vi "Smart_arm_Labview.vi"() -> ()   [LabVIEW 2022 SP3]
uses:
  <vilib>/Instr/_visa.llb/VISA Configure Serial Port (Instr).vi
panel:
  out "Number_of_runs":i16
  out "Stopped":bool
  out "Running":bool
  out "Read Target":string
  in  "Byte":u32
  in  "Joint 2":u8(knob) scale=45.0..100.0
  in  "Joint 1":u8(knob) scale=40.0..140.0
  in  "Buttom":u8(knob) scale=50.0..150.0
  out "Selected Mode":string
  in  "Mode_Selection":u8=1 max=2 step=1
  in  "Message Arduino -  Mode":bool
  in  "Claw":bool
  out "Previous settings of Claw, Buttom, Joint1, Joint2:":string
  in  "?":bool
  in  "Message Arduino - Angles":bool
  # "Smart Robotic Arm Control Panel"
  # "Automatic Mode"
  # "Select Mode"
  # "Hybrid Mode"
  # "[50° - 150°]"
  # "[40° - 140°]"
  # "Set Byte to 3  for Automatic mode\nOrtherwise set it to 0"
  # "0 - Manual\n             1 - Hybrid\n             2 - Automatic"
  # "[45° - 100°]"
  # "Open(0)"
  # "Close(1)"
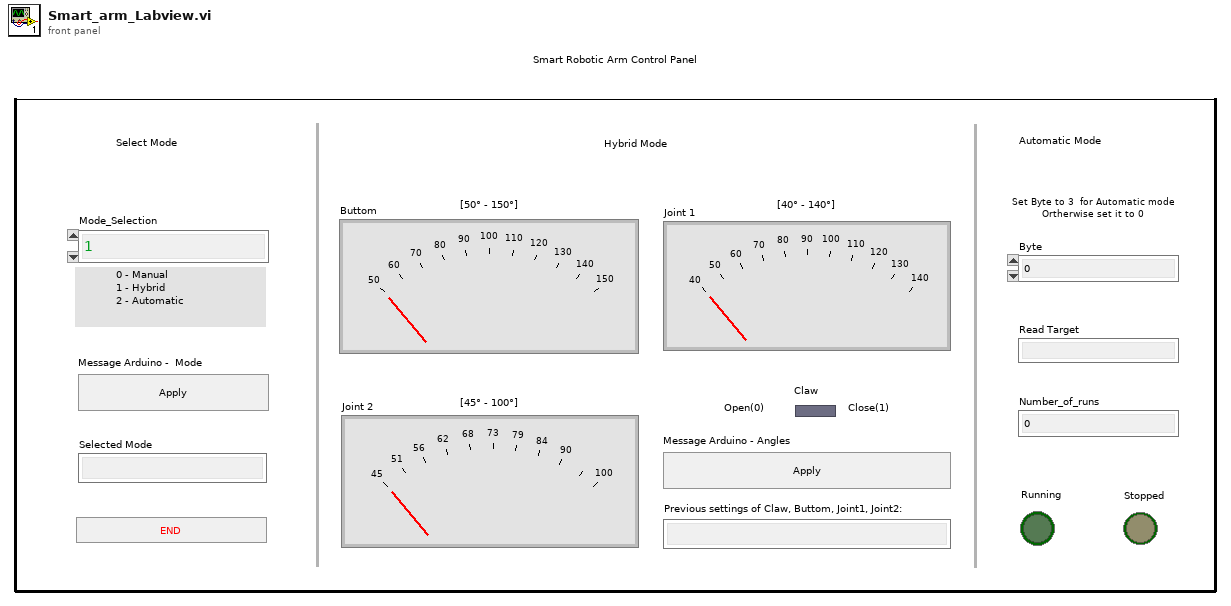
[diagram p1: front panel]
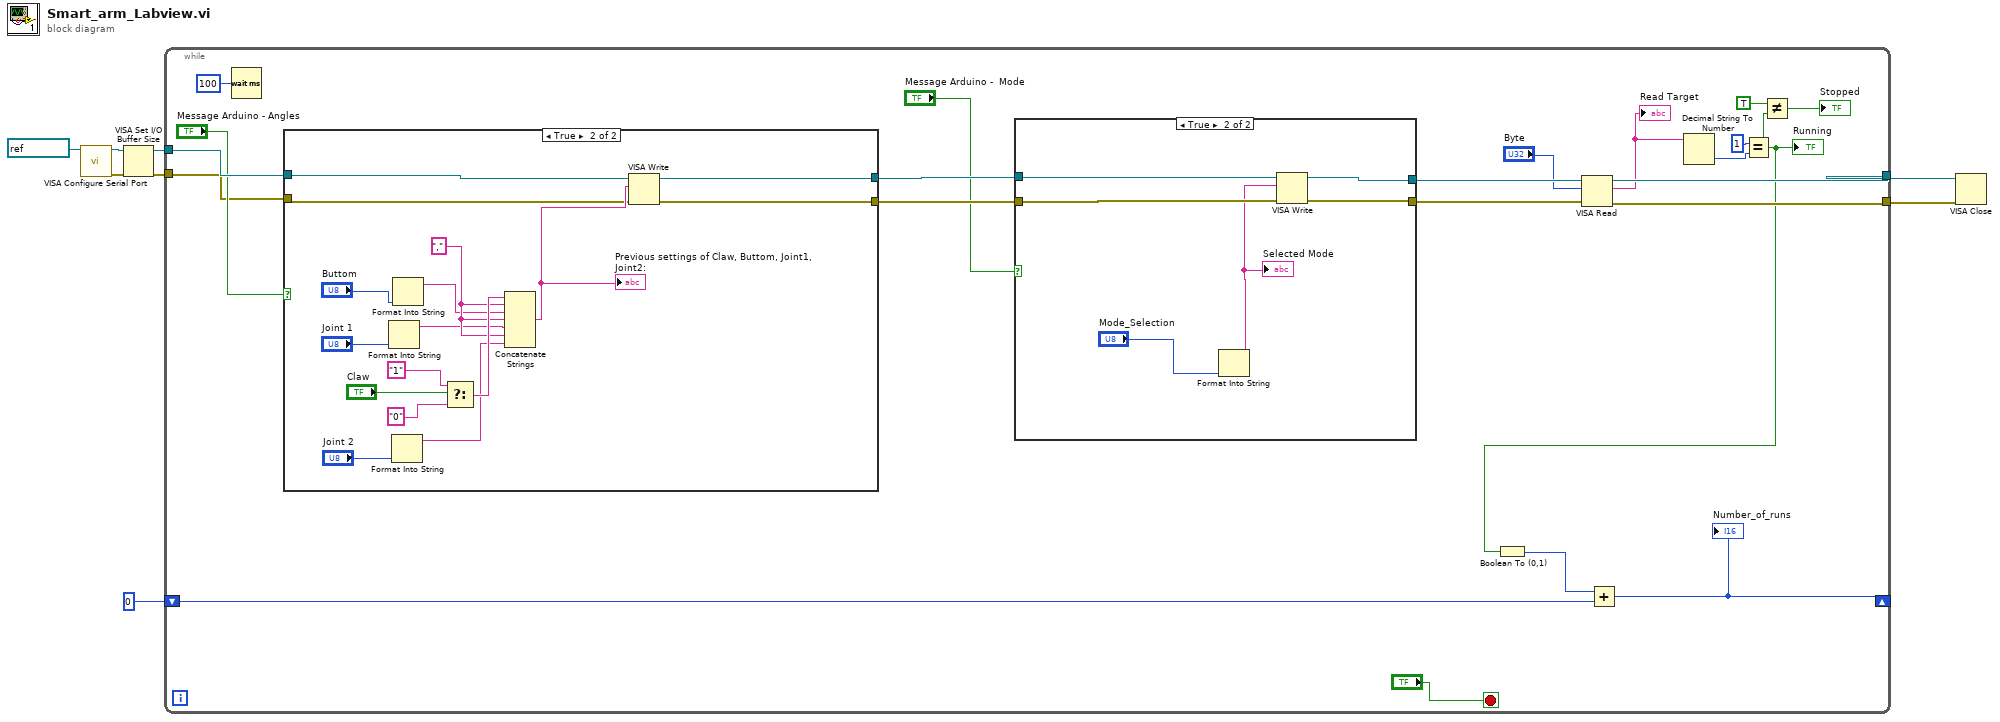
[diagram p0: block diagram]
diagram:
  n1 = call-poly "VISA Configure Serial Port"("VISA resource name"=refnum<visa-resource-name> "COM5") -> ("VISA resource name out"=w7:refnum<visa-resource-name>, "error out"=w6:errorcluster)  [unwired: 13 in]
  n2 = VISA Set I/O Buffer Size(VISA resource name=w7, error in (no error)=w6) -> (VISA resource name out=w5:refnum<visa-resource-name>, error out=w4:errorcluster)  [unwired: 2 in]
  n3 = while {
    tunnel: w5 -> [w29]
    tunnel: w4 -> [w27]
    tunnel: [w19] -> w3
    tunnel: [w20] -> w2
    shift-right: [w9] -> _
    shift-left: i16 0 -> [w10]
    stop <- "?" stop-if-true
    n4 = Wait (ms)(milliseconds to wait=u32 100) -> ()  [unwired: 1 out]
    n5 = case shown="True" "Message Arduino - Angles" {
      tunnel: [w40 w56] -> w26
      tunnel: [w39 w55] -> w25
      tunnel: w29 -> [w40 w54]
      tunnel: w27 -> [w39 w50]
      frame False {
      }
      frame True {
        w47 = ","
        n6 = Format Into String("Joint 1") -> (resulting string=w42:string)  [unwired: 3 in, 1 out]
        n7 = Format Into String("Joint 2") -> (resulting string=w41:string)  [unwired: 3 in, 1 out]
        n8 = Format Into String("Buttom") -> (resulting string=w45:string)  [unwired: 3 in, 1 out]
        n9 = Select(t="1", s="Claw", f="0") -> (s? t:f=w49:string)
        n10 = Concatenate Strings(w49, w47, w45, w47, w42, w47, w41) -> (w51:string)
        "Previous settings of Claw, Buttom, Joint1, Joint2:" <- w51
        n11 = VISA Write(VISA resource name=w54, write buffer=w51, error in (no error)=w50) -> (VISA resource name out=w56:refnum<visa-resource-name>, error out=w55:errorcluster)  [unwired: 1 out]
      }
    }
    n12 = case shown="True" "Message Arduino -  Mode" {
      tunnel: w26 -> [w32 w38]
      tunnel: w25 -> [w31 w35]
      tunnel: [w32 w37] -> w22
      tunnel: [w31 w36] -> w21
      frame False {
      }
      frame True {
        n13 = Format Into String("Mode_Selection") -> (resulting string=w33:string)  [unwired: 3 in, 1 out]
        "Selected Mode" <- w33
        n14 = VISA Write(VISA resource name=w38, write buffer=w33, error in (no error)=w35) -> (VISA resource name out=w37:refnum<visa-resource-name>, error out=w36:errorcluster)  [unwired: 1 out]
      }
    }
    n15 = VISA Read(VISA resource name=w22, byte count="Byte", error in (no error)=w21) -> (VISA resource name out=w19:refnum<visa-resource-name>, read buffer=w17:string, error out=w20:errorcluster)  [unwired: 1 out]
    "Read Target" <- w17
    n16 = Decimal String To Number(string=w17) -> (number=w15:i32)  [unwired: 2 in, 1 out]
    n17 = Equal?(x=1, y=w15) -> (x = y?=w12:bool)
    "Running" <- w12
    n18 = Boolean To (0,1)(Boolean=w12) -> (0, 1=w11:i16)
    n19 = Add(x=w11, y=w10) -> (x+y=w9:i16)
    "Number_of_runs" <- w9
    n20 = Not Equal?(x=TRUE, y=w12) -> (x != y?=→"Stopped":bool)
  }
  n21 = VISA Close(VISA resource name=w3, error in (no error)=w2) -> ()  [unwired: 1 out]
